vi "AIsFIFO_ECD.vi"   [LabVIEW 2017]
uses:
  <vilib>/rvi/DataTransferAndStorage/Container/Common/niFpgaContainerExecOnDevCompGetState.vi
  <vilib>/rvi/Emulation/niFpgaEmulationIsFPGAContextNoSignature.vi
  <vilib>/rvi/Emulation/niFpgaSctlEmulationGetInTimedLoop.vi
  <vilib>/rvi/errors/niFpgaSetErrorForExecOnDevCompSimple.vi
  <vilib>/rvi/eio/common/nirviEmuReportErrorAndStop.vi
  <vilib>/rvi/DataTransferAndStorage/Container/Common/niFpgaContainerGetUniqueNameForEmu.vi
  <vilib>/rvi/FIFO/Fifo_Resource/nirvififoEmulationSetSize.vi
  <vilib>/rvi/FIFO/Fifo_Resource/nirviFifoEmulationQueueMgr.vi
  <instcachedir>/0/nirviFifoEmulationQueueMgr_E5CAEC123FF24DC58D834DCA3CDAA9B5.lvgen/nirviFifoEmulationQueueMgr_E5CAEC123FF24DC58D834DCA3CDAA9B5_001.vi
  <vilib>/rvi/FIFO/Fifo_Resource/nirvififoEmulationDetermineInputValidOut.vi
  <vilib>/rvi/FIFO/Fifo_Resource/nirvififoEmulationCreateLock.vi
  <vilib>/rvi/Emulation/niFpgaProcessEmulError.vi
  <vilib>/rvi/FIFO/Fifo_Resource/nirvififoEmulationObtainLock.vi
  <vilib>/rvi/FIFO/Fifo_Resource/nirvififoEmulationReleaseLock.vi
  <vilib>/rvi/occurrence/nirviWaitOnOccurrenceBase.vi
  <vilib>/rvi/errors/nirviReportUnexpectedCaseInternalError.vi
  <vilib>/rvi/errors/nirviReportUnexpectedCaseInternalError (U32).vi
  <vilib>/Utility/error.llb/Clear Errors.vi
  <vilib>/rvi/interface/RandomDataEmulation/niFpgaRandomDataHandleErrors.vi
  <vilib>/rvi/eio/common/nirviEmuTemplateMethod_errors.vi
  <vilib>/rvi/DataTransferAndStorage/Container/XNode/niFpgaContainer.xnode
  <vilib>/rvi/FIFO/Fifo_Resource/niFpgaFifoEmulationRefIn.vi
  <vilib>/eio/EIONode/EIONode.xnode
diagram:
  w1 = fxp<+/-,26,5> -1.0 ("Element")
  w2 = fxp<+/-,26,5> -1.0 ("Element")
  n1 = xnode ("FIFO Method Node")("Element"=w2, "Timeout"=10, "FIFO (Eingang)"=refnum<k21> "FIFO" ("FIFO In")) -> ("FIFO (Ausgang)"=w224:refnum<k21>)  [unwired: 1 out]
  n2 = xnode ("FIFO Method Node")("Element"=w2, "Timeout"=10, "FIFO (Eingang)"=w224) -> ("FIFO (Ausgang)"=w222:refnum<k21>)  [unwired: 1 out]
  n3 = xnode ("FIFO Method Node")("Element"=w2, "Timeout"=10, "FIFO (Eingang)"=w222) -> ("FIFO (Ausgang)"=w220:refnum<k21>)  [unwired: 1 out]
  n4 = xnode ("FIFO Method Node")("Element"=w2, "Timeout"=10, "FIFO (Eingang)"=w220) -> ("FIFO (Ausgang)"=w218:refnum<k21>)  [unwired: 1 out]
  n5 = xnode ("FIFO Method Node")("Element"=w2, "Timeout"=10, "FIFO (Eingang)"=w218) -> ("FIFO (Ausgang)"=w216:refnum<k21>)  [unwired: 1 out]
  n6 = xnode ("FIFO Method Node")("Element"=w2, "Timeout"=10, "FIFO (Eingang)"=w216) -> ("FIFO (Ausgang)"=w214:refnum<k21>)  [unwired: 1 out]
  n7 = xnode ("FIFO Method Node")("Element"=w2, "Timeout"=10, "FIFO (Eingang)"=w214) -> ("FIFO (Ausgang)"=w212:refnum<k21>)  [unwired: 1 out]
  n8 = xnode ("FIFO Method Node")("Element"=w2, "Timeout"=10, "FIFO (Eingang)"=w212) -> ("FIFO (Ausgang)"=w210:refnum<k21>)  [unwired: 1 out]
  n9 = xnode ("FIFO Method Node")("Element"=w2, "Timeout"=10, "FIFO (Eingang)"=w210) -> ("FIFO (Ausgang)"=w208:refnum<k21>)  [unwired: 1 out]
  n10 = xnode ("FIFO Method Node")("Element"=w2, "Timeout"=10, "FIFO (Eingang)"=w208) -> ("FIFO (Ausgang)"=w206:refnum<k21>)  [unwired: 1 out]
  n11 = xnode ("FIFO Method Node")("Element"=w2, "Timeout"=10, "FIFO (Eingang)"=w206) -> ("FIFO (Ausgang)"=w204:refnum<k21>)  [unwired: 1 out]
  n12 = xnode ("FIFO Method Node")("Element"=w2, "Timeout"=10, "FIFO (Eingang)"=w204) -> ("FIFO (Ausgang)"=w202:refnum<k21>)  [unwired: 1 out]
  n13 = xnode ("FIFO Method Node")("Element"=w2, "Timeout"=10, "FIFO (Eingang)"=w202) -> ("FIFO (Ausgang)"=w200:refnum<k21>)  [unwired: 1 out]
  n14 = xnode ("FIFO Method Node")("Element"=w2, "Timeout"=10, "FIFO (Eingang)"=w200) -> ("FIFO (Ausgang)"=w198:refnum<k21>)  [unwired: 1 out]
  n15 = xnode ("FIFO Method Node")("Element"=w2, "Timeout"=10, "FIFO (Eingang)"=w198) -> ("FIFO (Ausgang)"=w196:refnum<k21>)  [unwired: 1 out]
  n16 = xnode ("FIFO Method Node")("Element"=w2, "Timeout"=10, "FIFO (Eingang)"=w196) -> ("FIFO (Ausgang)"=w194:refnum<k21>)  [unwired: 1 out]
  n17 = xnode ("FIFO Method Node")("Element"=w2, "Timeout"=10, "FIFO (Eingang)"=w194) -> ("FIFO (Ausgang)"=w192:refnum<k21>)  [unwired: 1 out]
  n18 = xnode ("FIFO Method Node")("Element"=w2, "Timeout"=10, "FIFO (Eingang)"=w192) -> ("FIFO (Ausgang)"=w190:refnum<k21>)  [unwired: 1 out]
  n19 = xnode ("FIFO Method Node")("Element"=w2, "Timeout"=10, "FIFO (Eingang)"=w190) -> ("FIFO (Ausgang)"=w188:refnum<k21>)  [unwired: 1 out]
  n20 = xnode ("FIFO Method Node")("Element"=w2, "Timeout"=10, "FIFO (Eingang)"=w188) -> ("FIFO (Ausgang)"=w186:refnum<k21>)  [unwired: 1 out]
  n21 = xnode ("FIFO Method Node")("Element"=w2, "Timeout"=10, "FIFO (Eingang)"=w186) -> ("FIFO (Ausgang)"=w184:refnum<k21>)  [unwired: 1 out]
  n22 = xnode ("FIFO Method Node")("Element"=w2, "Timeout"=10, "FIFO (Eingang)"=w184) -> ("FIFO (Ausgang)"=w182:refnum<k21>)  [unwired: 1 out]
  n23 = xnode ("FIFO Method Node")("Element"=w2, "Timeout"=10, "FIFO (Eingang)"=w182) -> ("FIFO (Ausgang)"=w180:refnum<k21>)  [unwired: 1 out]
  n24 = xnode ("FIFO Method Node")("Element"=w2, "Timeout"=10, "FIFO (Eingang)"=w180) -> ("FIFO (Ausgang)"=w178:refnum<k21>)  [unwired: 1 out]
  n25 = xnode ("FIFO Method Node")("Element"=w2, "Timeout"=10, "FIFO (Eingang)"=w178) -> ("FIFO (Ausgang)"=w176:refnum<k21>)  [unwired: 1 out]
  n26 = xnode ("FIFO Method Node")("Element"=w2, "Timeout"=10, "FIFO (Eingang)"=w176) -> ("FIFO (Ausgang)"=w174:refnum<k21>)  [unwired: 1 out]
  n27 = xnode ("FIFO Method Node")("Element"=w2, "Timeout"=10, "FIFO (Eingang)"=w174) -> ("FIFO (Ausgang)"=w172:refnum<k21>)  [unwired: 1 out]
  n28 = xnode ("FIFO Method Node")("Element"=w2, "Timeout"=10, "FIFO (Eingang)"=w172) -> ("FIFO (Ausgang)"=w170:refnum<k21>)  [unwired: 1 out]
  n29 = xnode ("FIFO Method Node")("Element"=w2, "Timeout"=10, "FIFO (Eingang)"=w170) -> ("FIFO (Ausgang)"=w168:refnum<k21>)  [unwired: 1 out]
  n30 = xnode ("FIFO Method Node")("Element"=w2, "Timeout"=10, "FIFO (Eingang)"=w168) -> ("FIFO (Ausgang)"=w166:refnum<k21>)  [unwired: 1 out]
  n31 = xnode ("FIFO Method Node")("Element"=w2, "Timeout"=10, "FIFO (Eingang)"=w166) -> ("FIFO (Ausgang)"=w164:refnum<k21>)  [unwired: 1 out]
  n32 = xnode ("FIFO Method Node")("Element"=w2, "Timeout"=10, "FIFO (Eingang)"=w164) -> ("FIFO (Ausgang)"=w67:refnum<k21>)  [unwired: 1 out]
  n33 = xnode "FPGA I/O Node"() -> ("Mod2/AI0"=w161:fxp<+/-,26,5>, "Mod2/AI1"=w158:fxp<+/-,26,5>, "Mod2/AI2"=w155:fxp<+/-,26,5>, "Mod2/AI3"=w153:fxp<+/-,26,5>, "Mod2/AI4"=w149:fxp<+/-,26,5>, "Mod2/AI5"=w146:fxp<+/-,26,5>, "Mod2/AI6"=w143:fxp<+/-,26,5>, "Mod2/AI7"=w140:fxp<+/-,26,5>, "Mod2/AI8"=w137:fxp<+/-,26,5>, "Mod2/AI9"=w134:fxp<+/-,26,5>, "Mod2/AI10"=w131:fxp<+/-,26,5>, "Mod2/AI11"=w128:fxp<+/-,26,5>, "Mod2/AI12"=w125:fxp<+/-,26,5>, "Mod2/AI13"=w122:fxp<+/-,26,5>, "Mod2/AI14"=w119:fxp<+/-,26,5>, "Mod2/AI15"=w116:fxp<+/-,26,5>, "Mod2/AI16"=w113:fxp<+/-,26,5>, "Mod2/AI17"=w110:fxp<+/-,26,5>, "Mod2/AI18"=w107:fxp<+/-,26,5>, "Mod2/AI19"=w104:fxp<+/-,26,5>, "Mod2/AI20"=w101:fxp<+/-,26,5>, "Mod2/AI21"=w98:fxp<+/-,26,5>, "Mod2/AI22"=w95:fxp<+/-,26,5>, "Mod2/AI23"=w92:fxp<+/-,26,5>, "Mod2/AI24"=w89:fxp<+/-,26,5>, "Mod2/AI25"=w86:fxp<+/-,26,5>, "Mod2/AI26"=w83:fxp<+/-,26,5>, "Mod2/AI27"=w80:fxp<+/-,26,5>, "Mod2/AI28"=w77:fxp<+/-,26,5>, "Mod2/AI29"=w74:fxp<+/-,26,5>, "Mod2/AI30"=w71:fxp<+/-,26,5>, "Mod2/AI31"=w68:fxp<+/-,26,5>)  [unwired: 32 in, 32 out]
  n34 = xnode ("FIFO Method Node")("Element"=w161, "Timeout"=10, "FIFO (Eingang)"=w67) -> ("FIFO (Ausgang)"=w159:refnum<k21>)  [unwired: 1 out]
  n35 = xnode ("FIFO Method Node")("Element"=w158, "Timeout"=10, "FIFO (Eingang)"=w159) -> ("FIFO (Ausgang)"=w156:refnum<k21>)  [unwired: 1 out]
  n36 = xnode ("FIFO Method Node")("Element"=w155, "Timeout"=10, "FIFO (Eingang)"=w156) -> ("FIFO (Ausgang)"=w152:refnum<k21>)  [unwired: 1 out]
  n37 = xnode ("FIFO Method Node")("Element"=w153, "Timeout"=10, "FIFO (Eingang)"=w152) -> ("FIFO (Ausgang)"=w150:refnum<k21>)  [unwired: 1 out]
  n38 = xnode ("FIFO Method Node")("Element"=w149, "Timeout"=10, "FIFO (Eingang)"=w150) -> ("FIFO (Ausgang)"=w147:refnum<k21>)  [unwired: 1 out]
  n39 = xnode ("FIFO Method Node")("Element"=w146, "Timeout"=10, "FIFO (Eingang)"=w147) -> ("FIFO (Ausgang)"=w144:refnum<k21>)  [unwired: 1 out]
  n40 = xnode ("FIFO Method Node")("Element"=w143, "Timeout"=10, "FIFO (Eingang)"=w144) -> ("FIFO (Ausgang)"=w141:refnum<k21>)  [unwired: 1 out]
  n41 = xnode ("FIFO Method Node")("Element"=w140, "Timeout"=10, "FIFO (Eingang)"=w141) -> ("FIFO (Ausgang)"=w138:refnum<k21>)  [unwired: 1 out]
  n42 = xnode ("FIFO Method Node")("Element"=w137, "Timeout"=10, "FIFO (Eingang)"=w138) -> ("FIFO (Ausgang)"=w135:refnum<k21>)  [unwired: 1 out]
  n43 = xnode ("FIFO Method Node")("Element"=w134, "Timeout"=10, "FIFO (Eingang)"=w135) -> ("FIFO (Ausgang)"=w132:refnum<k21>)  [unwired: 1 out]
  n44 = xnode ("FIFO Method Node")("Element"=w131, "Timeout"=10, "FIFO (Eingang)"=w132) -> ("FIFO (Ausgang)"=w129:refnum<k21>)  [unwired: 1 out]
  n45 = xnode ("FIFO Method Node")("Element"=w128, "Timeout"=10, "FIFO (Eingang)"=w129) -> ("FIFO (Ausgang)"=w126:refnum<k21>)  [unwired: 1 out]
  n46 = xnode ("FIFO Method Node")("Element"=w125, "Timeout"=10, "FIFO (Eingang)"=w126) -> ("FIFO (Ausgang)"=w123:refnum<k21>)  [unwired: 1 out]
  n47 = xnode ("FIFO Method Node")("Element"=w122, "Timeout"=10, "FIFO (Eingang)"=w123) -> ("FIFO (Ausgang)"=w120:refnum<k21>)  [unwired: 1 out]
  n48 = xnode ("FIFO Method Node")("Element"=w119, "Timeout"=10, "FIFO (Eingang)"=w120) -> ("FIFO (Ausgang)"=w117:refnum<k21>)  [unwired: 1 out]
  n49 = xnode ("FIFO Method Node")("Element"=w116, "Timeout"=10, "FIFO (Eingang)"=w117) -> ("FIFO (Ausgang)"=w114:refnum<k21>)  [unwired: 1 out]
  n50 = xnode ("FIFO Method Node")("Element"=w113, "Timeout"=10, "FIFO (Eingang)"=w114) -> ("FIFO (Ausgang)"=w111:refnum<k21>)  [unwired: 1 out]
  n51 = xnode ("FIFO Method Node")("Element"=w110, "Timeout"=10, "FIFO (Eingang)"=w111) -> ("FIFO (Ausgang)"=w108:refnum<k21>)  [unwired: 1 out]
  n52 = xnode ("FIFO Method Node")("Element"=w107, "Timeout"=10, "FIFO (Eingang)"=w108) -> ("FIFO (Ausgang)"=w105:refnum<k21>)  [unwired: 1 out]
  n53 = xnode ("FIFO Method Node")("Element"=w104, "Timeout"=10, "FIFO (Eingang)"=w105) -> ("FIFO (Ausgang)"=w102:refnum<k21>)  [unwired: 1 out]
  n54 = xnode ("FIFO Method Node")("Element"=w101, "Timeout"=10, "FIFO (Eingang)"=w102) -> ("FIFO (Ausgang)"=w99:refnum<k21>)  [unwired: 1 out]
  n55 = xnode ("FIFO Method Node")("Element"=w98, "Timeout"=10, "FIFO (Eingang)"=w99) -> ("FIFO (Ausgang)"=w96:refnum<k21>)  [unwired: 1 out]
  n56 = xnode ("FIFO Method Node")("Element"=w95, "Timeout"=10, "FIFO (Eingang)"=w96) -> ("FIFO (Ausgang)"=w93:refnum<k21>)  [unwired: 1 out]
  n57 = xnode ("FIFO Method Node")("Element"=w92, "Timeout"=10, "FIFO (Eingang)"=w93) -> ("FIFO (Ausgang)"=w90:refnum<k21>)  [unwired: 1 out]
  n58 = xnode ("FIFO Method Node")("Element"=w89, "Timeout"=10, "FIFO (Eingang)"=w90) -> ("FIFO (Ausgang)"=w87:refnum<k21>)  [unwired: 1 out]
  n59 = xnode ("FIFO Method Node")("Element"=w86, "Timeout"=10, "FIFO (Eingang)"=w87) -> ("FIFO (Ausgang)"=w84:refnum<k21>)  [unwired: 1 out]
  n60 = xnode ("FIFO Method Node")("Element"=w83, "Timeout"=10, "FIFO (Eingang)"=w84) -> ("FIFO (Ausgang)"=w81:refnum<k21>)  [unwired: 1 out]
  n61 = xnode ("FIFO Method Node")("Element"=w80, "Timeout"=10, "FIFO (Eingang)"=w81) -> ("FIFO (Ausgang)"=w78:refnum<k21>)  [unwired: 1 out]
  n62 = xnode ("FIFO Method Node")("Element"=w77, "Timeout"=10, "FIFO (Eingang)"=w78) -> ("FIFO (Ausgang)"=w75:refnum<k21>)  [unwired: 1 out]
  n63 = xnode ("FIFO Method Node")("Element"=w74, "Timeout"=10, "FIFO (Eingang)"=w75) -> ("FIFO (Ausgang)"=w72:refnum<k21>)  [unwired: 1 out]
  n64 = xnode ("FIFO Method Node")("Element"=w71, "Timeout"=10, "FIFO (Eingang)"=w72) -> ("FIFO (Ausgang)"=w69:refnum<k21>)  [unwired: 1 out]
  n65 = xnode ("FIFO Method Node")("Element"=w68, "Timeout"=10, "FIFO (Eingang)"=w69) -> ("FIFO (Ausgang)"=w3:refnum<k21>)  [unwired: 1 out]
  n66 = xnode ("FIFO Method Node")("Element"=w1, "Timeout"=10, "FIFO (Eingang)"=w3) -> ("FIFO (Ausgang)"=w64:refnum<k21>)  [unwired: 1 out]
  n67 = xnode ("FIFO Method Node")("Element"=w1, "Timeout"=10, "FIFO (Eingang)"=w64) -> ("FIFO (Ausgang)"=w62:refnum<k21>)  [unwired: 1 out]
  n68 = xnode ("FIFO Method Node")("Element"=w1, "Timeout"=10, "FIFO (Eingang)"=w62) -> ("FIFO (Ausgang)"=w60:refnum<k21>)  [unwired: 1 out]
  n69 = xnode ("FIFO Method Node")("Element"=w1, "Timeout"=10, "FIFO (Eingang)"=w60) -> ("FIFO (Ausgang)"=w58:refnum<k21>)  [unwired: 1 out]
  n70 = xnode ("FIFO Method Node")("Element"=w1, "Timeout"=10, "FIFO (Eingang)"=w58) -> ("FIFO (Ausgang)"=w56:refnum<k21>)  [unwired: 1 out]
  n71 = xnode ("FIFO Method Node")("Element"=w1, "Timeout"=10, "FIFO (Eingang)"=w56) -> ("FIFO (Ausgang)"=w54:refnum<k21>)  [unwired: 1 out]
  n72 = xnode ("FIFO Method Node")("Element"=w1, "Timeout"=10, "FIFO (Eingang)"=w54) -> ("FIFO (Ausgang)"=w52:refnum<k21>)  [unwired: 1 out]
  n73 = xnode ("FIFO Method Node")("Element"=w1, "Timeout"=10, "FIFO (Eingang)"=w52) -> ("FIFO (Ausgang)"=w50:refnum<k21>)  [unwired: 1 out]
  n74 = xnode ("FIFO Method Node")("Element"=w1, "Timeout"=10, "FIFO (Eingang)"=w50) -> ("FIFO (Ausgang)"=w48:refnum<k21>)  [unwired: 1 out]
  n75 = xnode ("FIFO Method Node")("Element"=w1, "Timeout"=10, "FIFO (Eingang)"=w48) -> ("FIFO (Ausgang)"=w46:refnum<k21>)  [unwired: 1 out]
  n76 = xnode ("FIFO Method Node")("Element"=w1, "Timeout"=10, "FIFO (Eingang)"=w46) -> ("FIFO (Ausgang)"=w44:refnum<k21>)  [unwired: 1 out]
  n77 = xnode ("FIFO Method Node")("Element"=w1, "Timeout"=10, "FIFO (Eingang)"=w44) -> ("FIFO (Ausgang)"=w42:refnum<k21>)  [unwired: 1 out]
  n78 = xnode ("FIFO Method Node")("Element"=w1, "Timeout"=10, "FIFO (Eingang)"=w42) -> ("FIFO (Ausgang)"=w40:refnum<k21>)  [unwired: 1 out]
  n79 = xnode ("FIFO Method Node")("Element"=w1, "Timeout"=10, "FIFO (Eingang)"=w40) -> ("FIFO (Ausgang)"=w38:refnum<k21>)  [unwired: 1 out]
  n80 = xnode ("FIFO Method Node")("Element"=w1, "Timeout"=10, "FIFO (Eingang)"=w38) -> ("FIFO (Ausgang)"=w36:refnum<k21>)  [unwired: 1 out]
  n81 = xnode ("FIFO Method Node")("Element"=w1, "Timeout"=10, "FIFO (Eingang)"=w36) -> ("FIFO (Ausgang)"=w34:refnum<k21>)  [unwired: 1 out]
  n82 = xnode ("FIFO Method Node")("Element"=w1, "Timeout"=10, "FIFO (Eingang)"=w34) -> ("FIFO (Ausgang)"=w32:refnum<k21>)  [unwired: 1 out]
  n83 = xnode ("FIFO Method Node")("Element"=w1, "Timeout"=10, "FIFO (Eingang)"=w32) -> ("FIFO (Ausgang)"=w30:refnum<k21>)  [unwired: 1 out]
  n84 = xnode ("FIFO Method Node")("Element"=w1, "Timeout"=10, "FIFO (Eingang)"=w30) -> ("FIFO (Ausgang)"=w28:refnum<k21>)  [unwired: 1 out]
  n85 = xnode ("FIFO Method Node")("Element"=w1, "Timeout"=10, "FIFO (Eingang)"=w28) -> ("FIFO (Ausgang)"=w26:refnum<k21>)  [unwired: 1 out]
  n86 = xnode ("FIFO Method Node")("Element"=w1, "Timeout"=10, "FIFO (Eingang)"=w26) -> ("FIFO (Ausgang)"=w24:refnum<k21>)  [unwired: 1 out]
  n87 = xnode ("FIFO Method Node")("Element"=w1, "Timeout"=10, "FIFO (Eingang)"=w24) -> ("FIFO (Ausgang)"=w22:refnum<k21>)  [unwired: 1 out]
  n88 = xnode ("FIFO Method Node")("Element"=w1, "Timeout"=10, "FIFO (Eingang)"=w22) -> ("FIFO (Ausgang)"=w20:refnum<k21>)  [unwired: 1 out]
  n89 = xnode ("FIFO Method Node")("Element"=w1, "Timeout"=10, "FIFO (Eingang)"=w20) -> ("FIFO (Ausgang)"=w18:refnum<k21>)  [unwired: 1 out]
  n90 = xnode ("FIFO Method Node")("Element"=w1, "Timeout"=10, "FIFO (Eingang)"=w18) -> ("FIFO (Ausgang)"=w16:refnum<k21>)  [unwired: 1 out]
  n91 = xnode ("FIFO Method Node")("Element"=w1, "Timeout"=10, "FIFO (Eingang)"=w16) -> ("FIFO (Ausgang)"=w14:refnum<k21>)  [unwired: 1 out]
  n92 = xnode ("FIFO Method Node")("Element"=w1, "Timeout"=10, "FIFO (Eingang)"=w14) -> ("FIFO (Ausgang)"=w12:refnum<k21>)  [unwired: 1 out]
  n93 = xnode ("FIFO Method Node")("Element"=w1, "Timeout"=10, "FIFO (Eingang)"=w12) -> ("FIFO (Ausgang)"=w10:refnum<k21>)  [unwired: 1 out]
  n94 = xnode ("FIFO Method Node")("Element"=w1, "Timeout"=10, "FIFO (Eingang)"=w10) -> ("FIFO (Ausgang)"=w8:refnum<k21>)  [unwired: 1 out]
  n95 = xnode ("FIFO Method Node")("Element"=w1, "Timeout"=10, "FIFO (Eingang)"=w8) -> ("FIFO (Ausgang)"=w6:refnum<k21>)  [unwired: 1 out]
  n96 = xnode ("FIFO Method Node")("Element"=w1, "Timeout"=10, "FIFO (Eingang)"=w6) -> ("FIFO (Ausgang)"=w4:refnum<k21>)  [unwired: 1 out]
  n97 = xnode ("FIFO Method Node")("Element"=w1, "Timeout"=10, "FIFO (Eingang)"=w4) -> ()  [unwired: 2 out]
